vi "ge_GXMLRcrsvParse.vi"(4 "String ID":string, 6 "File Item Contents":string, 7 "Empty XML Array?":bool, 8 "error in":errorcluster, 9 "Flat String In":string, 11 "Item TypeDesc":variant) -> (0 "error out":errorcluster, 1 "Flat String Out":string)   [LabVIEW 2012]
doc: "This recursive VI is the core engine responsible for searching the XML string. The VI recursively dives into the type definition cluster and identifies individual elements by name. In parallel the VI also looks at the XML string for tags that have the same name and hierarchy. If a match is found the data is extracted from the XML file and appropriately inserted into a flattened data string."
uses:
  <vilib>/Utility/VariantDataType/VariantType.lvlib
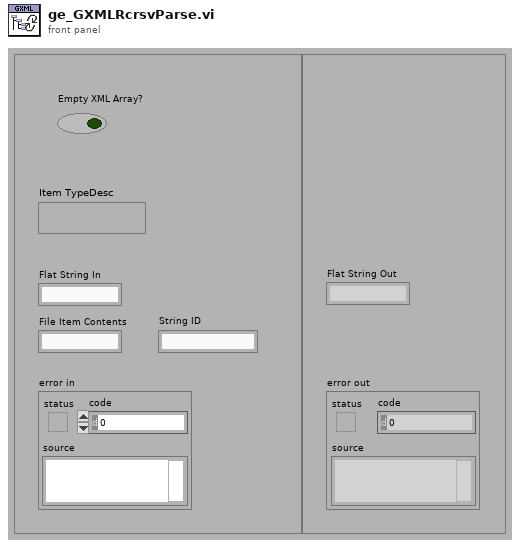
[diagram p1: front panel]
types:
  T1 = typedef "VariantType.lvlib/Type.ctl" = enum8{"Invalid Type", "Void", "I8", "I16", "I32", "I64", "U8", "U16", "U32", "U64", "Single Float", "Double Float", "Extended Float", "Single Complex", "Double Complex", "Extended Complex", "Enum U8", "Enum U16", "Enum U32", "Enum U64", "Single Float With Unit", "Double Float With Unit", "Extended Float With Unit", "Single Complex with Unit", "Double Complex with Unit", "Extended Complex with Unit", "Boolean", "String", "Path", "Picture", "Tag", "Array", "Cluster", "Variant", "LV Variant", "Waveform", "Timestamp", "Digital Waveform", "Digital Data", "ExpressData", "Refnum", "External Data", "VI", "Poly VI", "LabVIEW Class Instance", "Fixed Point"}
  T2 = cluster{"Item 'Name'":string, "Item Attributes":string, "Item Contents":string}
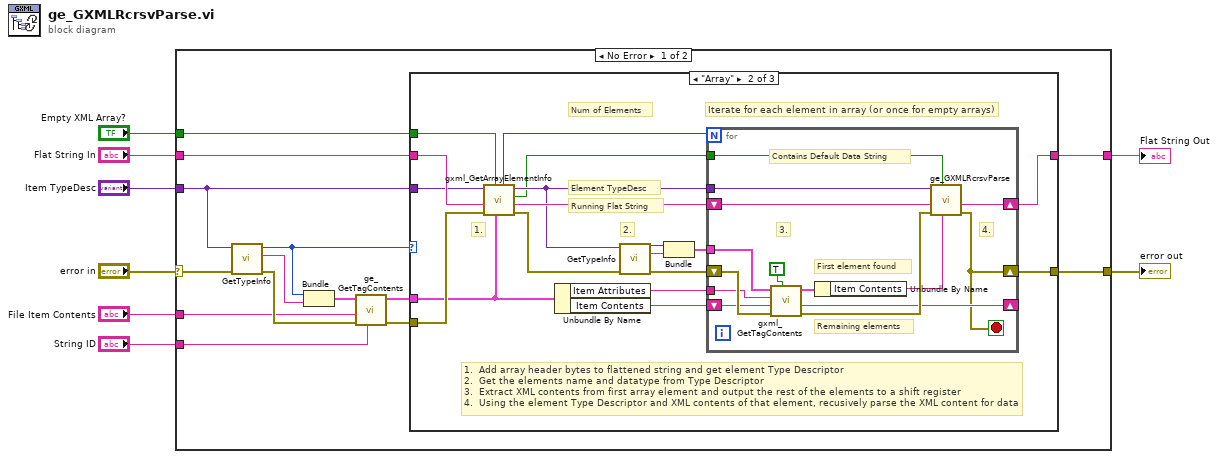
[diagram p0: block diagram]
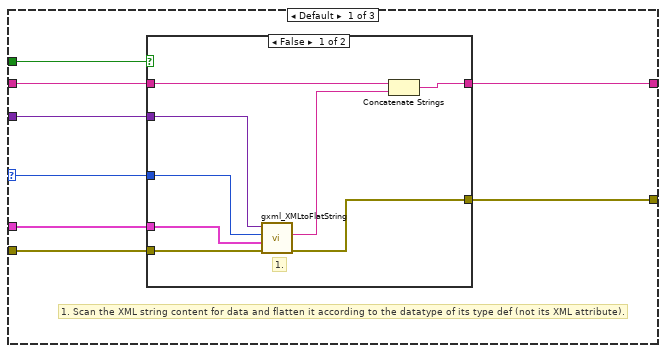
[diagram p2: hidden frame]
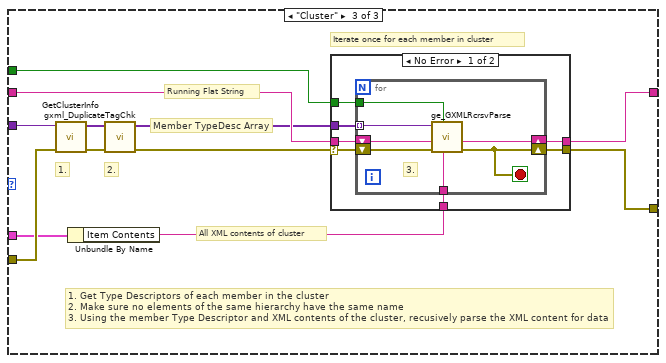
[diagram p4: hidden frame]
diagram:
  n1 = case shown="No Error" "error in" {
    selector: "error in" -> [w21 w102]
    tunnel: [w22 w102] -> w8
    tunnel: "File Item Contents" -> [w15 _]
    tunnel: "Item TypeDesc" -> [w20 _]
    tunnel: "Flat String In" -> [w11 w101]
    tunnel: [w19 w101] -> w4
    tunnel: "Empty XML Array?" -> [w10 _]
    tunnel: "String ID" -> [w9 _]
    frame No Error {
      n2 = call <vilib>:"GetTypeInfo.vi"("error in (no error)"=w21, "Variant"=w20) -> ("error out"=w18:errorcluster, "Name"=w12:string, "Type Enum"=w13:T1)  [unwired: 5 in, 2 out]
      n3 = Bundle("Type Enum"=w13, "Name"=w12) -> (w14:cluster{"Type Enum":T1, "Name":string})  [unwired: 1 in]
      n4 = call "ge_GetTagContents.vi"("String ID"=w9, "error in"=w18, "Item XML"=w15, "Item Name/Type"=w14) -> ("error out"=w17:errorcluster, "Item XML Data"=w16:T2)  [unwired: 5 in, 1 out]
      n5 = case shown="\"Array\"" w13 {
        selector: w13 -> [w28 _ _]
        tunnel: w20 -> [w29 w48 w84]
        tunnel: w17 -> [w30 w56 w83]
        tunnel: [w25 w57 w80] -> w22
        tunnel: w11 -> [w26 w51 w82]
        tunnel: [w24 w58 w81] -> w19
        tunnel: w16 -> [w27 w53 w79]
        tunnel: w10 -> [w23 w41 w77]
        frame Default {
          # "1. Scan the XML string content for data and flatten it according to the datatype of its type def (not its XML attribute)."
          n6 = case shown="False" w23 {
            tunnel: w30 -> [w38 w39]
            tunnel: w29 -> [w37 _]
            tunnel: w28 -> [w36 _]
            tunnel: w27 -> [w35 _]
            tunnel: w26 -> [w34 w40]
            tunnel: [w32 w39] -> w25
            tunnel: [w31 w40] -> w24
            frame False {
              # "1."
              n7 = call <userlib>:"gxml_XMLtoFlatString.vi"("error in"=w38, "Item XML Data"=w35, "Type Enum"=w36, "Item Type Desc"=w37) -> ("error out"=w32:errorcluster, "XML Data (Flat Str)"=w33:string)  [unwired: 6 in]
              n8 = Concatenate Strings(w34, w33) -> (w31:string)
            }
            frame True {
            }
          }
        }
        frame "Array" {
          # "Running Flat String"
          # "Element TypeDesc"
          # "Num of Elements"
          # "Iterate for each element in array (or once for empty arrays)"
          # "2."
          # "1."
          # "1.  Add array header bytes to flattened string and get element Type Descriptor\n2.  Get the elements name and datatype from Type Descriptor\n3.  Extract XML contents from first array element and output the rest of the elements to a shift register\n4.  Using the element Type Descriptor and XML contents of that element, recusively parse the XML content for data"
          n9 = call <userlib>:"gxml_GetArrayElementInfo.vi"("Item Data"=w53, "XML Array Empty?"=w41, "error in"=w56, "Flat String In"=w51, "Array TypeDesc"=w48) -> ("error out"=w50:errorcluster, "Flat String Out"=w52:string, "XML Array Empty?"=w42:bool, "Element TypeDesc"=w44:variant, "Element Count"=w43:i32)  [unwired: 2 in]
          n10 = Unbundle By Name(w53) -> ("Item Attributes"=w55:string, "Item Contents"=w54:string)
          n11 = call <vilib>:"GetTypeInfo.vi"("error in (no error)"=w50, "Variant"=w44) -> ("error out"=w49:errorcluster, "Name"=w46:string, "Type Enum"=w47:T1)  [unwired: 5 in, 2 out]
          n12 = Bundle("Type Enum"=w47, "Name"=w46) -> (w45:cluster{"Type Enum":T1, "Name":string})  [unwired: 1 in]
          n13 = for {
            N: w43 -> [_]
            tunnel: w44 -> [w61]
            shift-right: [w59] -> w58
            shift-left: w52 -> [w60]
            shift-right: [w69] -> _
            shift-left: w54 -> [w71]
            shift-right: [w68] -> w57
            shift-left: w49 -> [w72]
            tunnel: w55 -> [w67]
            tunnel: w45 -> [w63]
            tunnel: w42 -> [w62]
            stop <- w68 stop-if-true
            # "Contains Default Data String"
            # "Remaining elements"
            # "First element found"
            # "4."
            # "3."
            n14 = call <userlib>:"gxml_GetTagContents.vi"("Array Container?"=TRUE ("Include Tags?"), "error in"=w72, "Item XML"=w71, "Array Attributes"=w67, "Item Name/Type"=w63) -> ("error out"=w70:errorcluster, "XML After Closing Tag"=w69:string, "Item XML Data"=w65:T2)  [unwired: 4 in]
            n15 = Unbundle By Name(w65) -> ("Item Contents"=w64:string)
            n16 = call "ge_GXMLRcrsvParse.vi"("File Item Contents"=w64, "Empty XML Array?"=w62, "error in"=w70, "Flat String In"=w60, "Item TypeDesc"=w61) -> ("error out"=w68:errorcluster, "Flat String Out"=w59:string)  [unwired: 5 in]
          }
        }
        frame "Cluster" {
          # "2."
          # "Member TypeDesc Array"
          # "Running Flat String"
          # "All XML contents of cluster"
          # "Iterate once for each member in cluster"
          # "1."
          # "1. Get Type Descriptors of each member in the cluster\n2. Make sure no elements of the same hierarchy have the same name \n3. Using the member Type Descriptor and XML contents of the cluster, recusively parse the XML content for data"
          n17 = call <vilib>:"GetClusterInfo.vi"("error in (no error)"=w83, "Variant"=w84) -> ("error out"=w76:errorcluster, "Cluster Elements"=w74:variant[])  [unwired: 8 in]
          n18 = Unbundle By Name(w79) -> ("Item Contents"=w78:string)
          n19 = call <userlib>:"gxml_DuplicateTagChk.vi"("error in"=w76, "Cluster Elements"=w74) -> ("error out"=w75:errorcluster, "Cluster Elements Out"=w73:variant[])  [unwired: 7 in]
          n20 = case shown="No Error" w75 {
            selector: w75 -> [w86 w100]
            tunnel: w82 -> [w91 w99]
            tunnel: w73 -> [w90 _]
            tunnel: w78 -> [w89 _]
            tunnel: [w88 w99] -> w81
            tunnel: [w87 w100] -> w80
            tunnel: w77 -> [w85 _]
            frame No Error {
              n21 = for {
                shift-right: [w92] -> w88
                shift-left: w91 -> [w93]
                tunnel: w90 -> [w94] mode=indexing
                tunnel: w89 -> [w96]
                shift-right: [w97] -> w87
                shift-left: w86 -> [w98]
                tunnel: w85 -> [w95]
                stop <- w97 stop-if-true
                # "3."
                n22 = call "ge_GXMLRcrsvParse.vi"("File Item Contents"=w96, "Empty XML Array?"=w95, "error in"=w98, "Flat String In"=w93, "Item TypeDesc"=w94) -> ("error out"=w97:errorcluster, "Flat String Out"=w92:string)  [unwired: 5 in]
              }
            }
            frame Error {
            }
          }
        }
      }
    }
    frame Error {
    }
  }
  "error out" <- w8
  "Flat String Out" <- w4
